vi "detect device.vi"() -> ()   [LabVIEW 2019]
uses:
  <vilib>/nisyscfg/Close (System).vi
  <vilib>/nisyscfg/nisyscfg.lvlib
  <resource>/objmgr/niflexrioatomicsae.rc
  <resource>/objmgr/nicontrollersysapi.rc
panel:
  in  "Search Devices":string
  out "Table 2":string[][](table)
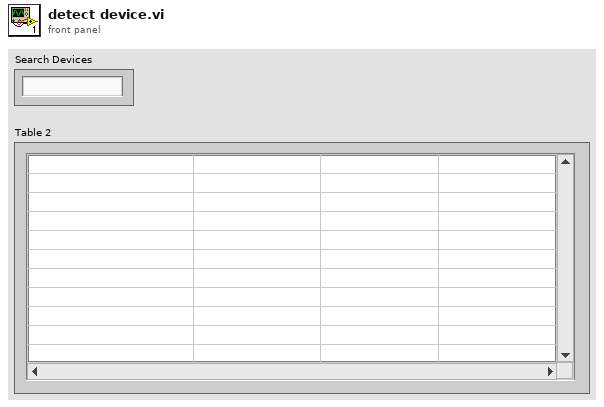
[diagram p1: front panel]
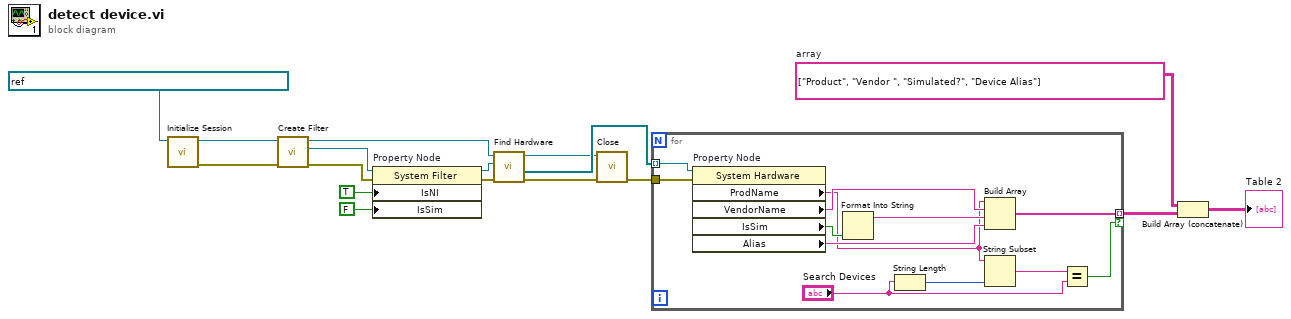
[diagram p0: block diagram]
diagram:
  w16 = string[][] [["Product", "Vendor ", "Simulated?", "Device Alias"]]  # array
  n1 = call <vilib>:"Initialize Session.vi"("Target (localhost)"=refnum<k21> "NI-PXIe8840QuadCore-2F266B38 (192.168.150.8)") -> ("error out"=w6:errorcluster, "Session out"=w5:refnum<k21>)  [unwired: 9 in]
  n2 = call <vilib>:"Create Filter.vi"("error in (no error)"=w6, "Session in"=w5) -> ("error out"=w3:errorcluster, "Filter out"=w4:refnum<k20>, "Session out"=w9:refnum<k21>)  [unwired: 7 in]
  n3 = property on="Property Node" class="System Filter"(reference=w4, error in=w3, "IsNI"=TRUE ("Devices & Chassis:Is NI Product"), "IsSim"=FALSE ("Devices & Chassis:Is Simulated")) -> (reference out=w8:refnum<k20>, error out=w7:errorcluster)
  n4 = call <vilib>:"Find Hardware.vi"("error in (no error)"=w7, "Filter in"=w8, "Session in"=w9) -> ("error out"=w11:errorcluster, "Resources out"=w13:refnum<k20>[], "Session out"=w12:refnum<k21>)  [unwired: 5 in, 1 out]
  n5 = call-poly <vilib>:"Close.vi"("error in (no error)"=w11, "Session in"=w12) -> ("error out"=w14:errorcluster)  [unwired: 9 in]
  n6 = for {
    tunnel: w13 -> [w28] mode=indexing
    tunnel: w14 -> [w29]
    tunnel: [w24] -> w15 mode=indexing if=w18
    n7 = property on="Property Node" class="System Hardware"(reference=w28, error in=w29) -> ("ProdName"=w20:string, "VendorName"=w26:string, "IsSim"=w27:bool, "Alias"=w23:string)  [unwired: 2 out]
    n8 = Format Into String "Format Into String"(w27) -> (resulting string=w25:string)  [unwired: 3 in, 1 out]
    n9 = String Length(string="Search Devices") -> (length=w21:i32)
    n10 = Build Array "Build Array"(w20, w26, w25, w23) -> (w24:string[])
    n11 = String Subset(string=w20, length (rest)=w21) -> (substring=w19:string)  [unwired: 1 in]
    n12 = Equal?(x=w19, y="Search Devices") -> (x = y?=w18:bool)
  }
  n13 = Build Array (concatenate) "Build Array"(w16, w15) -> (→"Table 2":string[][])
